vi "Sum_of_Three_Sines.vi"() -> ()   [LabVIEW 2022 SP3]
panel:
  out "Point Count":i32
  out "Waveform Graph":dbl[](graph)
  # "Sum_of_Three_Sines:"
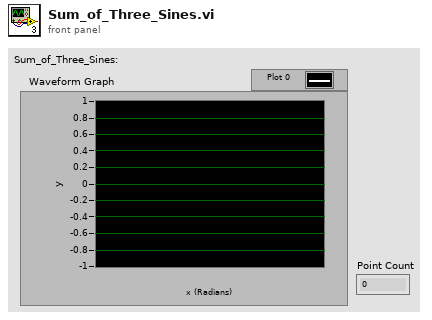
[diagram p1: front panel]
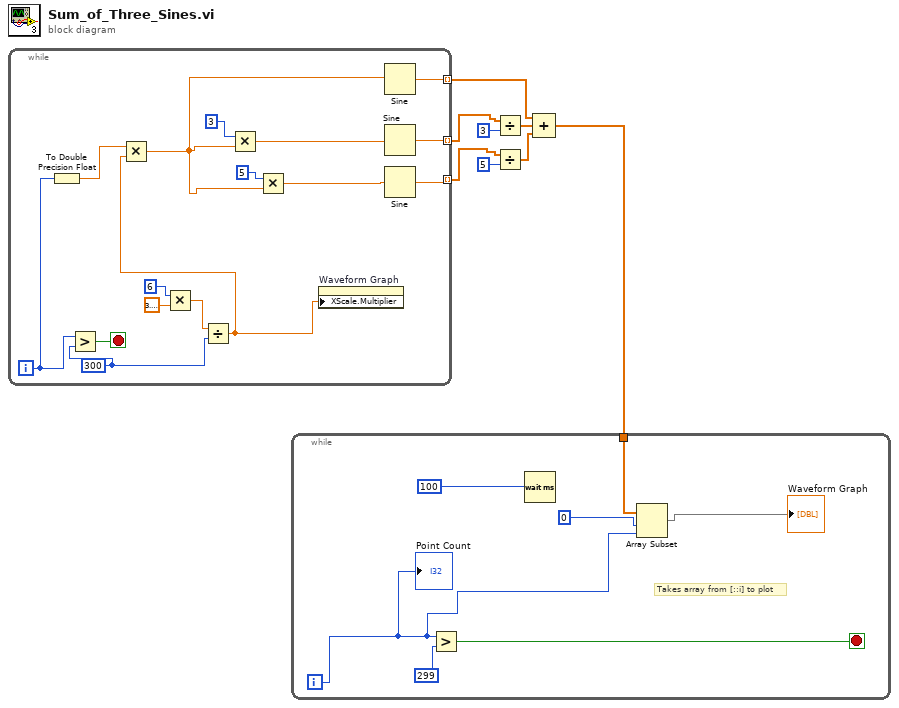
[diagram p0: block diagram]
diagram:
  n1 = while {
    tunnel: [w18] -> w4 mode=indexing
    tunnel: [w15] -> w7 mode=indexing
    tunnel: [w11] -> w6 mode=indexing
    i -> [w23]
    stop <- w24 stop-if-true
    w10 = 300
    n2 = To Double Precision Float(number=w23) -> (double precision float=w20:dbl)
    n3 = Greater?(x=w23, y=w10) -> (0:w24:bool)
    n4 = Multiply(x=6, y=3.141592653589793) -> (x*y=w9:dbl)
    n5 = Divide(x=w9, y=w10) -> (x/y=w19:dbl)
    n6 = Multiply(x=w20, y=w19) -> (x*y=w13:dbl)
    n7 = Multiply(x=3, y=w13) -> (x*y=w16:dbl)
    n8 = Multiply(x=5, y=w13) -> (x*y=w12:dbl)
    n9 = property on="Waveform Graph" class="WFGraph (strict)"("XScale.Multiplier"=w19) -> ()  [unwired: 2 in, 2 out]
    n10 = Sine(x=w13) -> (sin(x)=w18:dbl)
    n11 = Sine(x=w16) -> (sin(x)=w15:dbl)
    n12 = Sine(x=w12) -> (sin(x)=w11:dbl)
  }
  n13 = Divide(x=w7, y=3) -> (x/y=w3:dbl[])
  n14 = Divide(x=w6, y=5) -> (x/y=w2:dbl[])
  n15 = Compound Arithmetic op=ADD(w4, w3, w2) -> (w1:dbl[])
  n16 = while {
    tunnel: w1 -> [w28]
    i -> [w26]
    stop <- w30 stop-if-true
    # "Takes array from [::i] to plot"
    n17 = Greater?(x=w26, y=299) -> (0:w30:bool)
    n18 = Wait (ms)(milliseconds to wait=100 ("Point Waittime  (ms)")) -> ()  [unwired: 1 out]
    n19 = Array Subset(array=w28, index=0, length=w26) -> (→"Waveform Graph":dbl[])
    "Point Count" <- w26
  }
